vi "Change File Extension.vi"(10 "New Extension (Txt)":string="txt", 11 "Path In":path) -> (2 "Previous Extension":string, 3 "Path Out":path)   [LabVIEW 2017, in "lvcsm File Support.lvlib"]
uses:
  lvcsm File Support.lvlib
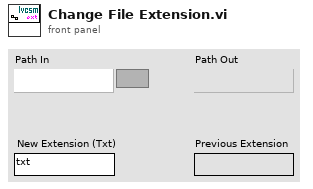
[diagram p1: front panel]
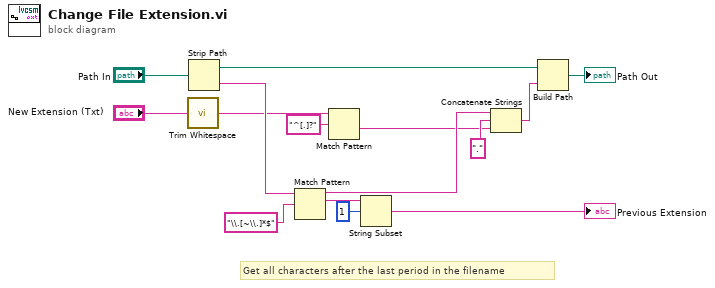
[diagram p0: block diagram]
diagram:
  # "Get all characters after the last period in the filename"
  n1 = call <vilib>:"Trim Whitespace.vi"("string"="New Extension (Txt)") -> ("trimmed string"=w1:string)  [unwired: 1 in]
  n2 = Strip Path(path="Path In") -> (stripped path=w9:path, name=w6:string)
  n3 = Match Pattern(string=w6, regular expression="\\.[~\\.]*$") -> (before substring=w10:string, match substring=w8:string)  [unwired: 3 out]
  n4 = Match Pattern(string=w1, regular expression="^[.]?") -> (after substring=w2:string)  [unwired: 4 out]
  n5 = String Subset(string=w8, offset (0)=1) -> (substring=→"Previous Extension":string)  [unwired: 1 out]
  n6 = Concatenate Strings(w10, "." ("string"), w2) -> (w11:string)
  n7 = Build Path(base path=w9, name or relative path=w11) -> (appended path=→"Path Out":path)
